vi "Create File.vi"(8 "error in":errorcluster, 11 "TDMS in":refnum<class "TDMS.lvclass">) -> (0 "error out":errorcluster, 3 "TDMS out":refnum<class "TDMS.lvclass">)   [LabVIEW 2017, in "Report_lib.lvlib" / "TDMS.lvclass"]
doc: "This method create or replace TDMS file\nwith defined FilePath and set in it \nTDMS global properties"
uses:
  TDMS.lvclass
  TDMS.lvclass/TDMS.ctl
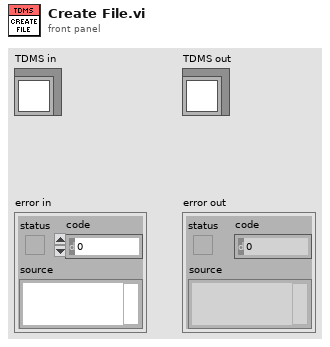
[diagram p1: front panel]
types:
  T1 = enum16{"open", "open or create", "create or replace", "create", "open (read-only)"}
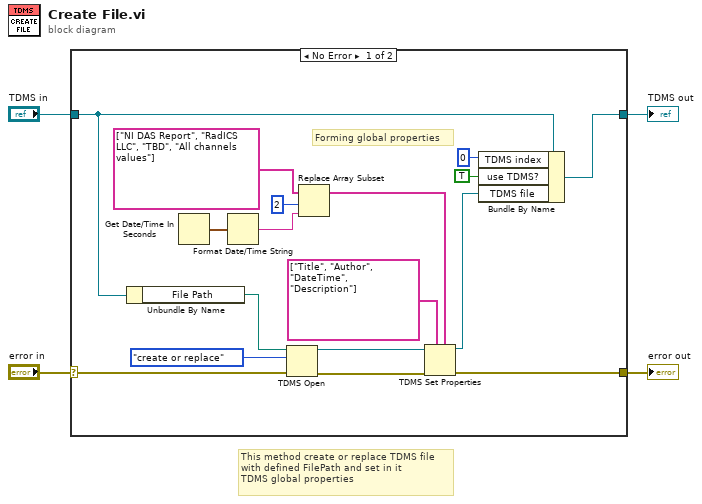
[diagram p0: block diagram]
diagram:
  # "This method create or replace TDMS file\nwith defined FilePath and set in it \nTDMS global properties"
  n1 = case shown="No Error" "error in" {
    selector: "error in" -> [w13 w23]
    tunnel: [w12 w23] -> w3
    tunnel: [w6 w22] -> w1
    tunnel: "TDMS in" -> [w7 w22]
    frame No Error {
      # "Forming global properties"
      n2 = Unbundle By Name(w7) -> ("File Path"=w14:path)
      n3 = Get Date/Time In Seconds() -> (seconds since 1Jan1904=w17:timestamp)
      n4 = Format Date/Time String(seconds (now)=w17) -> (date/time string=w10:string)  [unwired: 2 in]
      n5 = TDMS Open(8:w13, 10:T1."create or replace" ("operation (0:open)"), 11:w14) -> (0:w21:errorcluster, 3:w20:refnum<k34>)  [unwired: 4 in]
      n6 = Replace Array Subset(array=string[] ["NI DAS Report", "RadICS LLC", "TBD", "All channels values"], new element=w10, index=2) -> (w15:string[])
      n7 = TDMS Set Properties(5:w15, 7:string[] ["Title", "Author", "DateTime", "Description"], 8:w21, 11:w20) -> (0:w12:errorcluster, 3:w5:refnum<k34>)  [unwired: 2 in, 2 out]
      n8 = Bundle By Name(cluster=w7, "TDMS index"=0, "use TDMS?"=TRUE, "TDMS file"=w5) -> (w6:refnum<class "TDMS.lvclass">)
    }
    frame Error {
    }
  }
  "error out" <- w3
  "TDMS out" <- w1
